vi "generate channels from UI.vi"(8 "error in":errorcluster, 11 "VI Refnum":refnum<vi>) -> (0 "error out":errorcluster, 3 "channels":refnum<class "TBM channel.lvclass">[](array[class]))   [LabVIEW 2015, in "UI Reference configuration.lvclass"]
uses:
  UI Reference configuration.lvclass
  <vilib>/NI/Tag Bus Module Framework/channel/TBM channel.lvclass
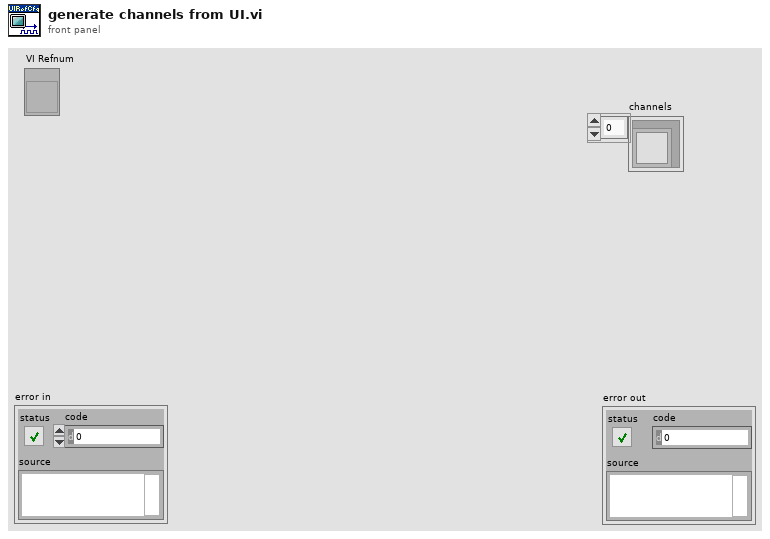
[diagram p1: front panel]
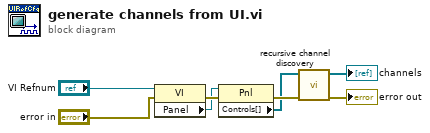
[diagram p0: block diagram]
diagram:
  n1 = property class="VI"(reference="VI Refnum", error in="error in") -> (error out=w8:errorcluster, "Panel"=w7:refnum<vi>)  [unwired: 1 out]
  n2 = property class="Pnl"(reference=w7, error in=w8) -> (error out=w6:errorcluster, "Controls[]"=w5:refnum<vi>[])  [unwired: 1 out]
  n3 = call "recursive channel discovery.vi"("error in (no error)"=w6, "Controls[]"=w5) -> ("error out"=→"error out":errorcluster, "Array"=→"channels":refnum<class "TBM channel.lvclass">[])  [unwired: 8 in]
